vi "Configure Desired Output State.vi"(8 "error in (no error)":errorcluster, 9 "output state (Constant Voltage)":i32(ring) items=["Constant Voltage"=0, "Constant Current"=1, "Unregulated"=4, "Over Voltage"=2, "Over Current"=3], 10 "channel name (\"CHANNEL1\")":string="CHANNEL1", 11 "CS++DCPwr in":refnum<class "CS++DCPwr.lvclass">) -> (0 "error out":errorcluster, 2 "in state":bool, 3 "CS++DCPwr out":refnum<class "CS++DCPwr.lvclass">)   [LabVIEW 2016, in "CS++DCPwr.lvlib" / "CS++DCPwr.lvclass"]
doc: "This VI returns whether the power supply is in a particular output state.\n\nA constant voltage condition occurs when the output voltage is equal to the value of the IviDCPwr>>Basic Operation>>Voltage Level property and the current is less than or equal to the value of the IviDCPwr>>Basic Operation>>Current Limit property.\n\nA constant current condition occurs when the output current is equal to the value of the IviDCPwr>>Basic Operation>>Current Limit property and the IviDCPwr>>Basic Operation>>Current Limit Behavior property is set to IVIDCPWR_VAL_CURRENT_REGULATE.\n\nAn unregulated condition occurs when the output voltage is less than the value of the IviDCPwr>>Basic Operation>>Voltage Level property and the current is less than the value of the IviDCPwr>>Basic Operation>>Current Limit property.\n\nAn over-voltage condition occurs when the output voltage is equal to or greater than the value of the IviDCPwr>>Basic Operation>>OVP Limit property and the IviDCPwr>>Basic Operation>>OVP Enabled property is set to TRUE.\n\nAn over-current condition occurs when the output current is equal to or greater than the value of the IviDCPwr>>Basic Operation>>Current Limit property and the IviDCPwr>>Basic Operation>>Current Limit Behavior property is set to IVIDCPWR_VAL_CURRENT_TRIP. \n\nWhen either an over-voltage condition or an over-current condition occurs, the power supply's output protection disables the output. If the power supply is in an over-voltage or over-current state, it does not produce power until the output protection is reset. The IviDCPwr Reset Output Protection VI resets the output protection. Once the output protection is reset, the power supply resumes generating a power signal."
uses:
  CS++DCPwr.lvclass
  CSPP_Core/Classes/CS++ProcessVariables/ProcessVariable/PV.lvclass
  PV-Enum.ctl
  CSPP_Core/Classes/CS++ProcessVariables/ProcessVariable/PV.lvclass/PV.ctl
  CS++DCPwr.lvclass/CS++DCPwr.ctl
  CSPP_Core/Classes/CS++ProcessVariables/ProcessVariable/Write Data.vi
  CSPP_Core/Classes/CS++ProcessVariables/ProcessVariable/Write Timestamp.vi
  CSPP_Core/Classes/CS++ProcessVariables/ProcessVariable/Write Quality.vi
  CSPP_Core/Classes/CS++ProcessVariables/ProcessVariable/Write status.vi
  CSPP_Core/Classes/CS++ProcessVariables/PVConnection/PVConnection.lvclass
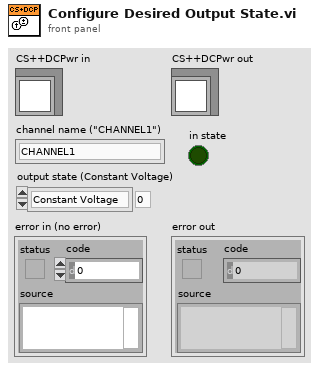
[diagram p1: front panel]
types:
  T1 = typedef "CS++DCPwr.lvlib/CS++DCPwr.lvclass/PV-Enum.ctl" = enum16{"CurrentLimit", "MaxCurrentLimit", "MaxVoltageLevel", "Measure-A", "Measure-V", "OVPLimit", "Range", "TriggerCurrentLimit", "TriggerVoltageLevel", "VoltageLevel", "Behavior", "DesiredOutputState", "RangeType", "TriggerSource", "InState", "OutputEnable", "OVPEnabled"}
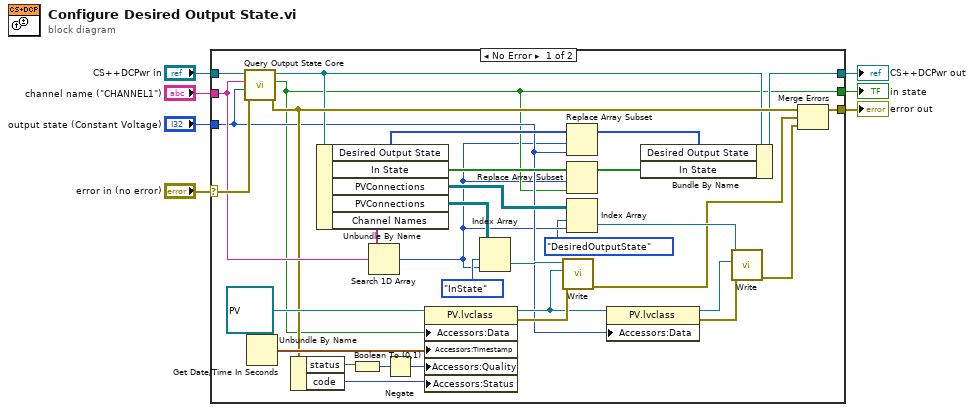
[diagram p0: block diagram]
diagram:
  n1 = case shown="No Error" "error in (no error)" {
    selector: "error in (no error)" -> [w39 w42]
    tunnel: [w31 w42] -> w6
    tunnel: [w22 w41] -> w4
    tunnel: "CS++DCPwr in" -> [w40 w41]
    tunnel: "channel name (\"CHANNEL1\")" -> [w34 _]
    tunnel: "output state (Constant Voltage)" -> [w14 _]
    tunnel: [w11 _] -> w1
    frame No Error {
      n2 = call-dynamic "Query Output State Core.vi"("error in (no error)"=w39, "output state (Constant Voltage)"=w14, "channel name (\"CHANNEL1\")"=w34, "CS++DCPwr in"=w40) -> ("error out"=w26:errorcluster, "in state"=w11:bool, "CS++DCPwr out"=w23:refnum<class "CS++DCPwr.lvclass">)  [unwired: 5 in]
      n3 = Get Date/Time In Seconds() -> (seconds since 1Jan1904=w38:timestamp)
      n4 = Unbundle By Name(w26) -> ("status"=w30:bool, "code"=w28:i32)
      n5 = Unbundle By Name(w23) -> ("Desired Output State"=w21:i32[], "In State"=w25:bool[], "PVConnections"=w16:refnum<class "PVConnection.lvclass">[][], "PVConnections"=w33:refnum<class "PVConnection.lvclass">[][], "Channel Names"=w35:string[])
      n6 = Boolean To (0,1)(Boolean=w30) -> (0, 1=w29:i16)
      n7 = Search 1D Array(1D array=w35, element=w34) -> (index of element=w9:i32)  [unwired: 1 in]
      n8 = Negate(x=w29) -> (-x=w27:i16)
      n9 = property class="PV.lvclass"(reference=refnum<class "PV.lvclass"> refnum ("PV"), "Accessors:Data"=w11, "Accessors:Timestamp"=w38, "Accessors:Quality"=w27, "Accessors:Status"=w28) -> (reference out=w15:refnum<class "PV.lvclass">, error out=w36:errorcluster)  [unwired: 1 in]
      n10 = Index Array(array=w33, index (row)=PV-Enum."InState" ("PV-Enum"), index (col)=w9) -> (element=w32:refnum<class "PVConnection.lvclass">)
      n11 = call "Write.vi"("error in (no error)"=w36, "PV"=w15, "PVConnection in"=w32) -> ("error out"=w13:errorcluster)  [unwired: 7 in, 1 out]
      n12 = Replace Array Subset(array=w21, new element=w14, index=w9) -> (w20:i32[])
      n13 = Replace Array Subset(array=w25, new element=w11, index=w9) -> (w24:bool[])
      n14 = Index Array(array=w16, index (row)=PV-Enum."DesiredOutputState" ("PV-Enum"), index (col)=w9) -> (element=w19:refnum<class "PVConnection.lvclass">)
      n15 = property class="PV.lvclass"(reference=w15, "Accessors:Data"=w14) -> (reference out=w18:refnum<class "PV.lvclass">, error out=w17:errorcluster)  [unwired: 1 in]
      n16 = Bundle By Name(cluster=w23, "Desired Output State"=w20, "In State"=w24) -> (w22:refnum<class "CS++DCPwr.lvclass">)
      n17 = call "Write.vi"("error in (no error)"=w17, "PV"=w18, "PVConnection in"=w19) -> ("error out"=w12:errorcluster)  [unwired: 7 in, 1 out]
      n18 = Merge Errors(w26, w13, w12) -> (w31:errorcluster)
    }
    frame Error {
    }
  }
  "error out" <- w6
  "CS++DCPwr out" <- w4
  "in state" <- w1
